vi "TEST - LVOOP Return Class Name.vi"(8 "error in (no error)":errorcluster) -> (0 "error out":errorcluster, 2 "Pass":bool)   [LabVIEW 2020, in "test_openg_variant.lvlib"]
uses:
  test_openg_variant.lvlib
  LVOOP Data/Class 1/Class 1.lvclass
  <vilib>/addons/_JKI Toolkits/Caraya/classes/Assert/Assert True.vi
  source/library/openg_variant.lvlib
  <vilib>/addons/_JKI Toolkits/Caraya/classes/Test/Test.lvclass
  <vilib>/addons/_JKI Toolkits/Caraya/classes/Assert/Assert.lvclass
panel:
  out "Test Name":string
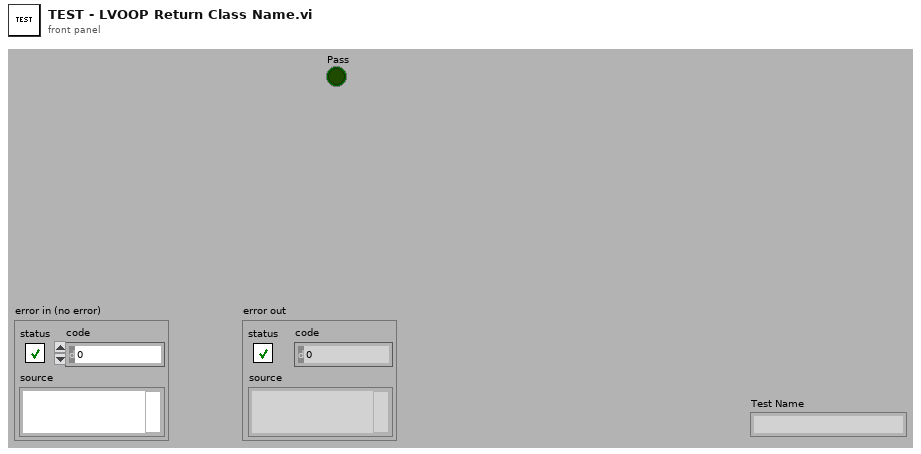
[diagram p1: front panel]
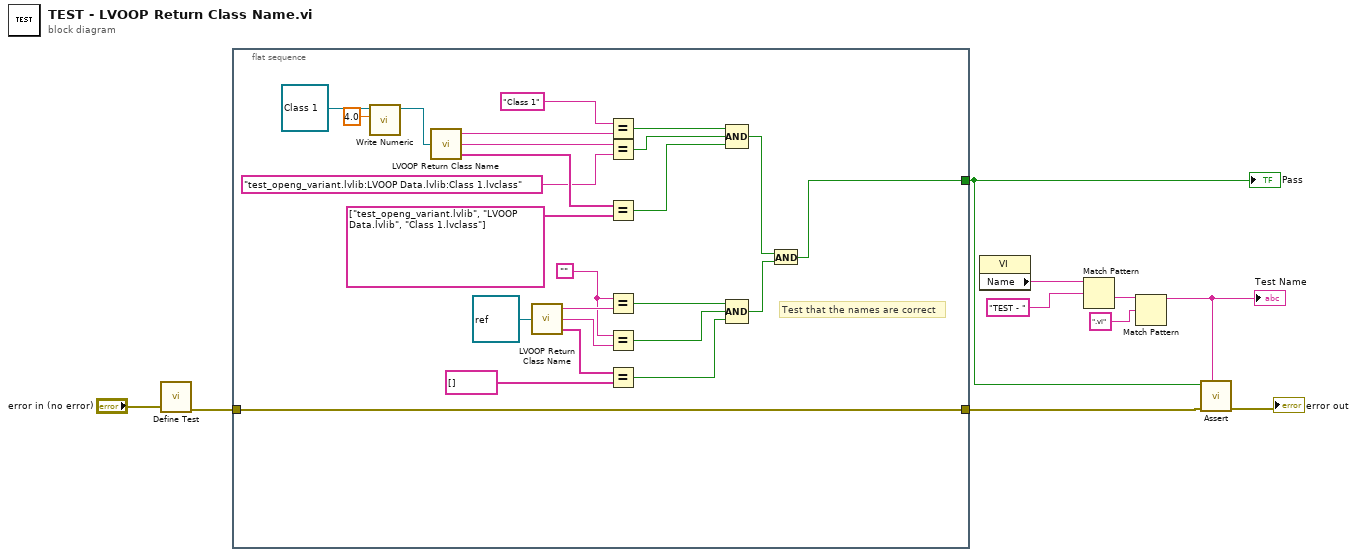
[diagram p0: block diagram]
diagram:
  n1 = call <vilib>:"Define Test.vi"("error in (no error)"="error in (no error)") -> ("error out"=w1:errorcluster)  [unwired: 9 in, 1 out]
  n2 = flat-sequence {
    tunnel: [w12] -> w5
    tunnel: [w11] -> w2
    tunnel: w1 -> [w11]
    frame #0 {
      w30 = ""
      # "Test that the names are correct"
      n3 = call "Write Numeric.vi"("Numeric"=4.0, "Class 1 in"=refnum<class "Class 1.lvclass"> refnum) -> ("Class 1 out"=w15:refnum<class "Class 1.lvclass">)  [unwired: 9 in]
      n4 = call "LVOOP Return Class Name.vi"("Object"=w15) -> ("Class Base Name"=w35:string, "Qualified Name"=w18:string, "Qualified Name Array"=w24:string[])
      n5 = call "LVOOP Return Class Name.vi"("Object"=refnum<class> refnum) -> ("Class Base Name"=w32:string, "Qualified Name"=w31:string, "Qualified Name Array"=w28:string[])
      n6 = Equal?(x="Class 1", y=w35) -> (x = y?=w21:bool)
      n7 = Equal?(x=w18, y="test_openg_variant.lvlib:LVOOP Data.lvlib:Class 1.lvclass" ("Fully Qualified Name")) -> (x = y?=w17:bool)
      n8 = Equal?(x=w24, y=string[] ["test_openg_variant.lvlib", "LVOOP Data.lvlib", "Class 1.lvclass"] ("Qualified Name Array")) -> (x = y?=w16:bool)
      n9 = Equal?(x=w30, y=w32) -> (x = y?=w25:bool)
      n10 = Equal?(x=w30, y=w31) -> (x = y?=w26:bool)
      n11 = Equal?(x=w28, y=string[] [] ("Qualified Name Array")) -> (x = y?=w27:bool)
      n12 = Compound Arithmetic op=AND(w21, w17, w16) -> (w20:bool)
      n13 = Compound Arithmetic op=AND(w25, w26, w27) -> (w19:bool)
      n14 = And(x=w20, y=w19) -> (x .and. y?=w12:bool)
    }
  }
  n15 = property class="VI"() -> ("Name"=w9:string)  [unwired: 2 in, 2 out]
  n16 = Match Pattern(string=w9, regular expression="TEST - ") -> (after substring=w10:string)  [unwired: 1 in, 3 out]
  n17 = Match Pattern(string=w10, regular expression=".vi") -> (before substring=w6:string)  [unwired: 1 in, 3 out]
  "Test Name" <- w6
  n18 = call-poly <vilib>:"Assert.vi"("Label"=w6, "error in (no error)"=w2, "True?"=w5) -> ("error out"=→"error out":errorcluster)  [unwired: 7 in, 1 out]
  "Pass" <- w5
